vi "AnalogIn_read.vi"(8 "error in (no error)":errorcluster, 11 "mbed_LVLibrary.lvlib:AnalogIn.lvclass":refnum<class "AnalogIn.lvclass">) -> (0 "error out":errorcluster, 2 "value":dbl, 3 "mbed_LVLibrary.lvlib:AnalogIn.lvclass 2":refnum<class "AnalogIn.lvclass">)   [LabVIEW 2011, in "mbed_LVLibrary.lvlib" / "AnalogIn.lvclass"]
uses:
  AnalogIn.lvclass
  AnalogIn.lvclass/AnalogIn.ctl
  Transport Mechanisms/mbed/mbed.lvclass
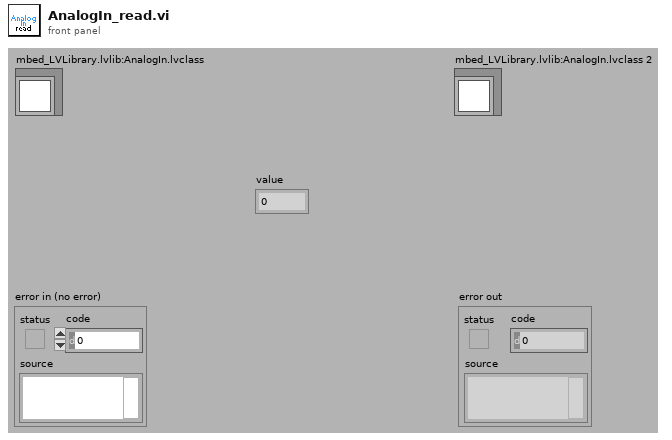
[diagram p1: front panel]
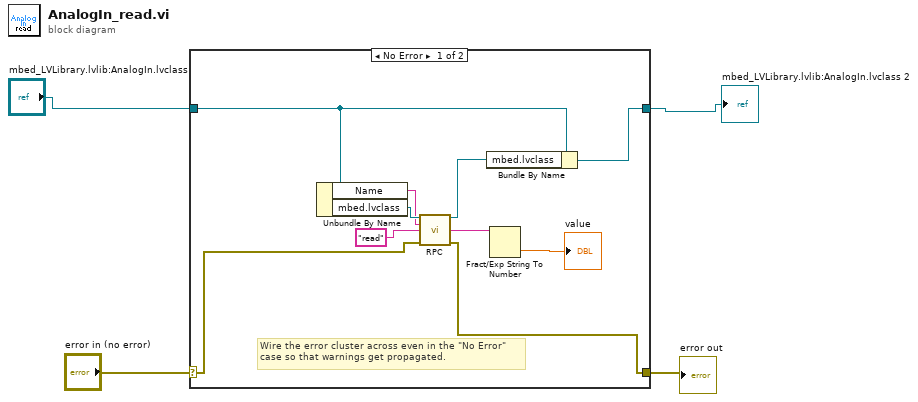
[diagram p0: block diagram]
diagram:
  n1 = case shown="No Error" "error in (no error)" {
    selector: "error in (no error)" -> [w6 w16]
    tunnel: [w5 w16] -> w3
    tunnel: [w8 w15] -> w1
    tunnel: "mbed_LVLibrary.lvlib:AnalogIn.lvclass" -> [w9 w15]
    frame No Error {
      # "Wire the error cluster across even in the \"No Error\"\ncase so that warnings get propagated."
      n2 = Unbundle By Name(w9) -> ("Name"=w12:string, "mbed.lvclass"=w14:refnum<class "mbed.lvclass">)
      n3 = call-dynamic "RPC.vi"("mbed in"=w14, "Name"=w12, "method"="read", "error in (no error)"=w6) -> ("mbed out"=w7:refnum<class "mbed.lvclass">, "RPC Result"=w11:string, "error out"=w5:errorcluster)  [unwired: 9 in]
      n4 = Bundle By Name(cluster=w9, "mbed.lvclass"=w7) -> (w8:refnum<class "AnalogIn.lvclass">)
      n5 = Fract/Exp String To Number(string=w11) -> (number=→"value":dbl)  [unwired: 3 in, 1 out]
    }
    frame Error {
    }
  }
  "error out" <- w3
  "mbed_LVLibrary.lvlib:AnalogIn.lvclass 2" <- w1
